vi "Math to Center (SubVI).vi"(9 "R Horizontal Image Resolution":dbl=320.0, 10 "N Width Of Target (Pixels)":dbl=39.0, 11 "Pixels To Center":dbl) -> (0 "Target Found Out":bool, 1 "Degrees To Center (Degree) Out":dbl, 2 "Distance To Target (Inches) Out":dbl, 3 "Distance To Center (Inches) Out":dbl)   [LabVIEW 2017, in "VisionSystem.lvlib"]
uses:
  VisionSystem.lvlib
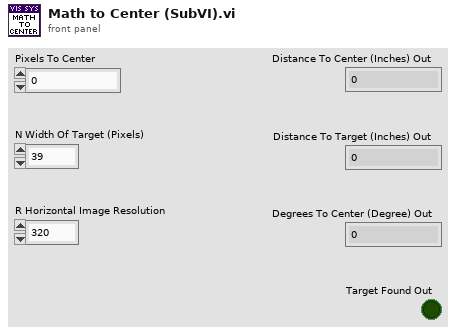
[diagram p1: front panel]
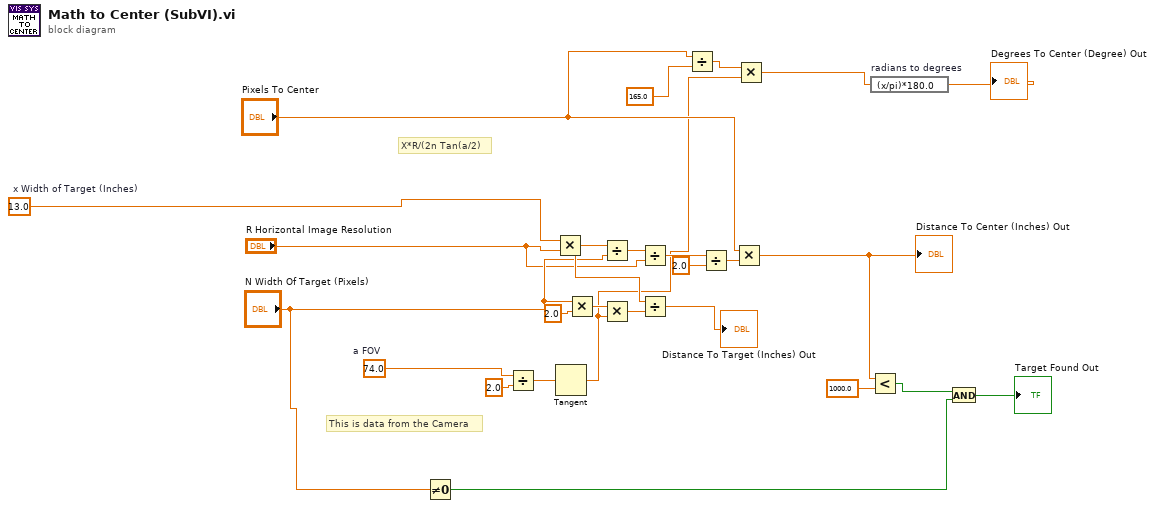
[diagram p0: block diagram]
diagram:
  w12 = 13.0  # x Width of Target (Inches)
  w22 = 74.0  # a FOV
  # "This is data from the Camera"
  # "X*R/(2n Tan(a/2)"
  n1 = Not Equal To 0?(x="N Width Of Target (Pixels)") -> (x != 0?=w13:bool)
  n2 = Divide(x=w22, y=2.0) -> (x/y=w8:dbl)
  n3 = Multiply(x=w12, y="R Horizontal Image Resolution") -> (x*y=w21:dbl)
  n4 = Tangent(1:w8) -> (0:w3:dbl)
  n5 = Multiply(x="N Width Of Target (Pixels)", y=2.0) -> (x*y=w24:dbl)
  n6 = Divide(x=w21, y="N Width Of Target (Pixels)") -> (x/y=w20:dbl)
  n7 = Multiply(x=w24, y=w3) -> (x*y=w23:dbl)
  n8 = Divide(x=w20, y="R Horizontal Image Resolution") -> (x/y=w19:dbl)
  n9 = Divide(x=w21, y=w23) -> (x/y=→"Distance To Target (Inches) Out":dbl)
  n10 = Divide(x="Pixels To Center", y=165.0) -> (x/y=w4:dbl)
  n11 = Divide(x=w19, y=2.0) -> (x/y=w9:dbl)
  n12 = Multiply(x="Pixels To Center", y=w9) -> (x*y=w18:dbl)
  "Distance To Center (Inches) Out" <- w18
  n13 = Multiply(x=w4, y=w3) -> (x*y=w2:dbl)
  n14 = Less?(x=w18, y=1000.0) -> (x < y?=w14:bool)
  n15 = expression code="(x/pi)*180.0" "radians to degrees"(w2) -> (→"Degrees To Center (Degree) Out":dbl)
  n16 = And(x=w14, y=w13) -> (x .and. y?=→"Target Found Out":bool)
